vi "Create Map Attribute.vi"(9 "Attribute":string, 10 "Map Attribute":T1, 11 "Root Attributes In":map{string, string}(c390)) -> (3 "Root Attributes":map{string, string}(c390))   [LabVIEW 2020, in "Panther Dashboard.lvlib" / "Project.lvclass"]
uses:
  Project.lvclass
  Panther Dashboard/Map Attribute--enum.ctl
  Panther Dashboard/Panther Dashboard.lvlib
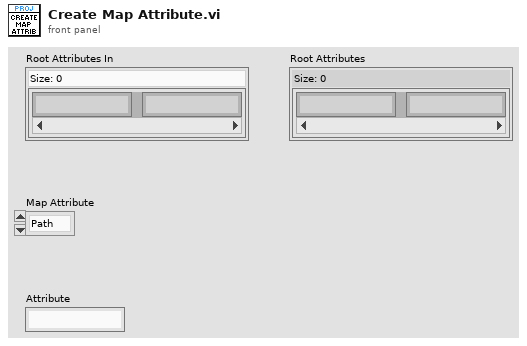
[diagram p1: front panel]
types:
  T1 = typedef "Panther Dashboard.lvlib/Map Attribute--enum.ctl" = enum16{"Path", "ModuleType", "Module Description", "Dependency?", "Target"}
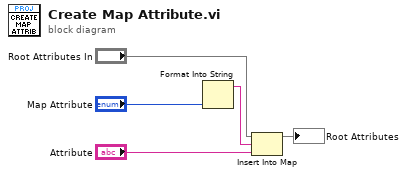
[diagram p0: block diagram]
diagram:
  n1 = Format Into String("Map Attribute") -> (resulting string=w2:string)  [unwired: 3 in, 1 out]
  n2 = Insert Into Map(map in="Root Attributes In", key=w2, value="Attribute") -> (map out=→"Root Attributes":map{string, string})  [unwired: 2 out]
